vi "mu.vi"(5 "y^n":dbl=1.0 format="%#_13g", 7 "x^n":dbl=1.0 format="%#_13g", 9 "Array":u32[][](array[numeric]), 10 "cy":u16, 11 "cx":u16) -> (3 "sum":dbl)   [LabVIEW 2021]
uses:
  <vilib>/picture/picture.llb/Draw True-Color Pixmap.vi
panel:
  out "multiplicado":picture
  out "elementos":picture
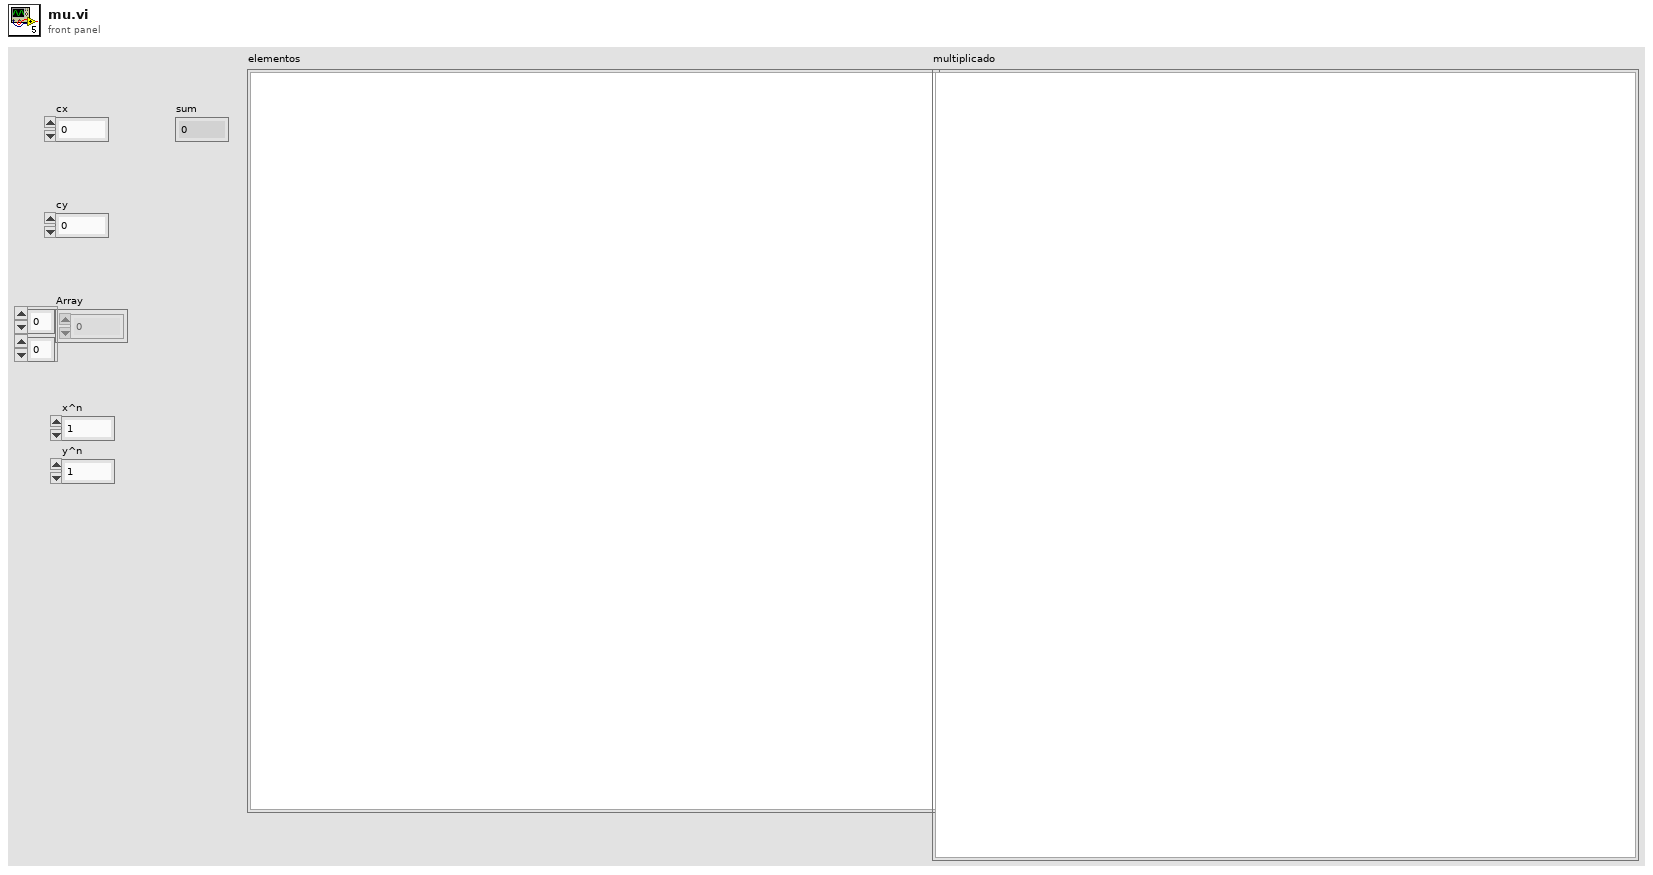
[diagram p1: front panel]
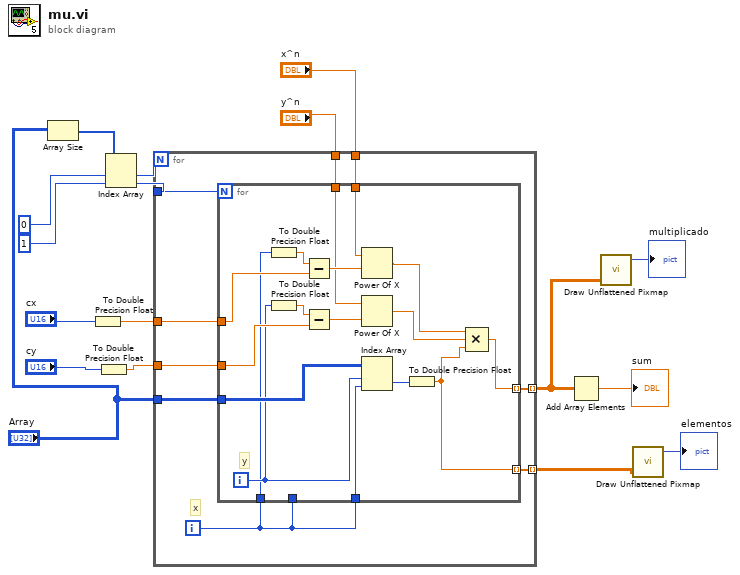
[diagram p0: block diagram]
diagram:
  n1 = Array Size(array="Array") -> (size(s)=w8:i32[])
  n2 = To Double Precision Float(number="cx") -> (double precision float=w17:dbl)
  n3 = To Double Precision Float(number="cy") -> (double precision float=w14:dbl)
  n4 = Index Array(array=w8, index #1=0 ("index"), index #2=1 ("index")) -> (element #1=w9:i32, element #2=w10:i32)
  n5 = for {
    N: w9 -> [_]
    tunnel: "Array" -> [w26]
    tunnel: w14 -> [w25]
    tunnel: w10 -> [w24]
    tunnel: [w23] -> w2 mode=indexing
    tunnel: "x^n" -> [w22]
    tunnel: "y^n" -> [w21]
    tunnel: w17 -> [w20]
    tunnel: [w18] -> w5 mode=indexing
    i -> [w19]
    # "x"
    n6 = for {
      N: w24 -> [_]
      tunnel: w26 -> [w37]
      tunnel: w25 -> [w33]
      tunnel: w19 -> [w39]
      tunnel: w19 -> [_]
      tunnel: [w36] -> w23 mode=indexing
      tunnel: w22 -> [w35]
      tunnel: w21 -> [w34]
      tunnel: w20 -> [w32]
      tunnel: w19 -> [w28]
      tunnel: [w27] -> w18 mode=indexing
      i -> [w29]
      # "y"
      n7 = To Double Precision Float(number=w28) -> (double precision float=w31:dbl)
      n8 = To Double Precision Float(number=w29) -> (double precision float=w30:dbl)
      n9 = Subtract(x=w31, y=w32) -> (x-y=w43:dbl)
      n10 = Subtract(x=w30, y=w33) -> (x-y=w42:dbl)
      n11 = Power Of X(1:w43, 2:w35) -> (0:w41:dbl)
      n12 = Power Of X(1:w42, 2:w34) -> (0:w40:dbl)
      n13 = Index Array(array=w37, index (row)=w29, index (col)=w39) -> (element=w38:u32)
      n14 = To Double Precision Float(number=w38) -> (double precision float=w27:dbl)
      n15 = Compound Arithmetic op=MULTIPLY(w41, w40, w27) -> (w36:dbl)
    }
  }
  n16 = Add Array Elements(numeric array=w2) -> (sum=→"sum":dbl)
  n17 = call-poly <vilib>:"Draw Unflattened Pixmap.vi"("data (RGB format)"=w2) -> ("new picture"=→"multiplicado":picture)  [unwired: 8 in]
  n18 = call-poly <vilib>:"Draw Unflattened Pixmap.vi"("data (RGB format)"=w5) -> ("new picture"=→"elementos":picture)  [unwired: 8 in]
